vi "ColorAPI_Quit.vi"(8 "错误输入（无错误）":errorcluster) -> (0 "错误输出":errorcluster)   [LabVIEW 2011, in "ColorSensorlib.lvlib"]
uses:
  ColorSensorlib.lvlib
  ColorDis.dll
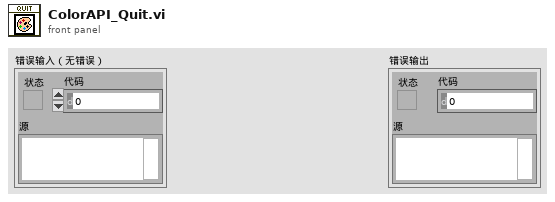
[diagram p1: front panel]
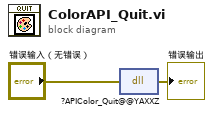
[diagram p0: block diagram]
diagram:
  n1 = dll-call lib="PTH1Cabs D\tDocumentsDesktop颜色传感器LabViewColorDis.dll" fn="?APIColor_Quit@@YAXXZ"(error in="错误输入（无错误）") -> (error out=→"错误输出":errorcluster)  [unwired: 3 in, 1 out]
